vi "Check SLAM LM's.vi"(8 "error in (no error)":errorcluster, 10 "SLAM In":T2, 11 "Observed LM Array":T1(array[cluster])) -> (0 "error out":errorcluster, 2 "SLAM Out":T2, 3 "Observed LM Out":T1(array[cluster]))   [LabVIEW 2009]
uses:
  Controls/SLAM.ctl
  <vilib>/Analysis/Matrix/Datatypes/RealMatrix.ctl
  <vilib>/Analysis/Matrix/NI_Matrix.lvlib
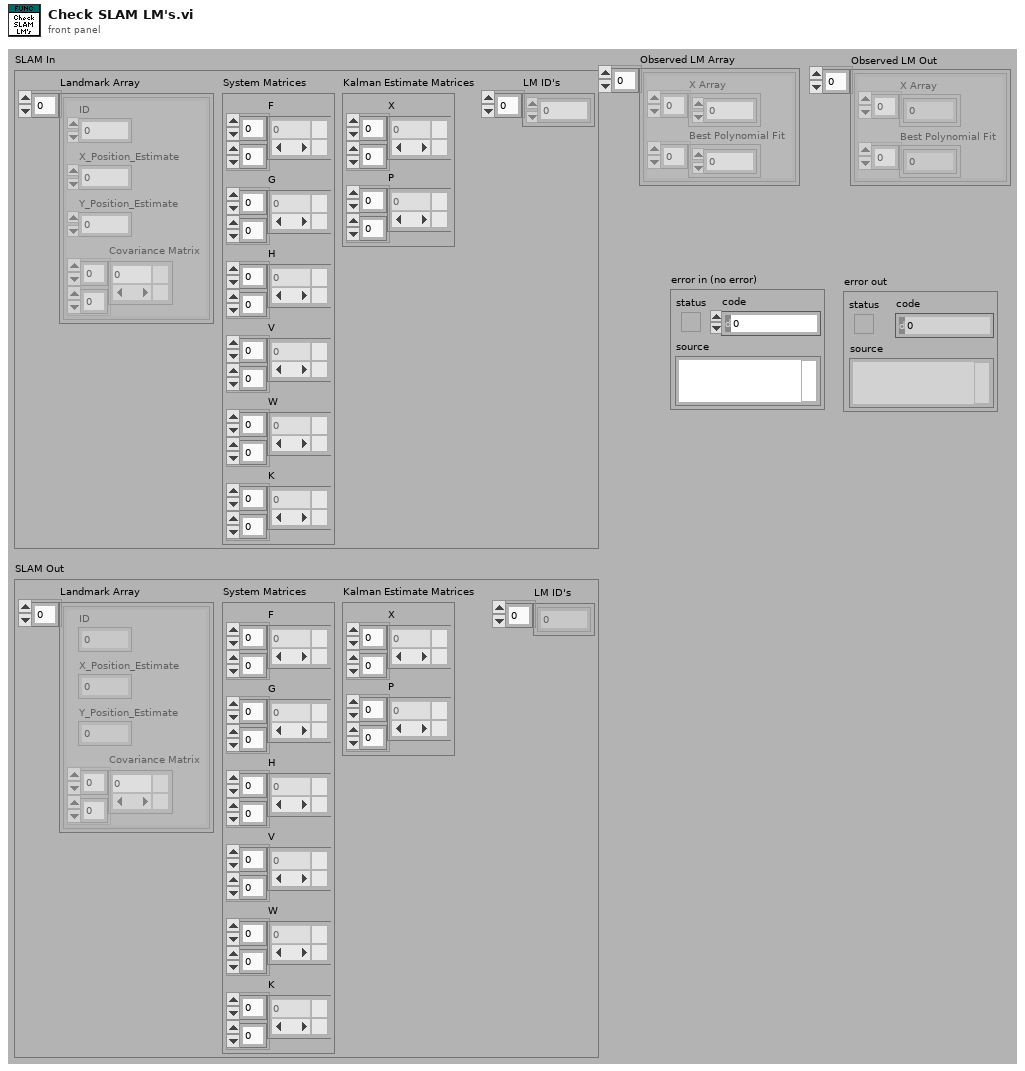
[diagram p1: front panel]
types:
  T1 = cluster{"X Array":dbl[], "Best Polynomial Fit":dbl[]}[]
  T2 = typedef "SLAM.ctl" = cluster{"Landmark Array":cluster{"ID":dbl, "X_Position_Estimate":dbl, "Y_Position_Estimate":dbl, "Covariance Matrix":T3}[], "System Matrices":cluster{"F":T3, "G":T3, "H":T3, "V":T3, "W":T3, "K":T3}, "Kalman Estimate Matrices":cluster{"X":T3, "P":T3}, "LM ID's":dbl[]}
  T3 = typedef "NI_Matrix.lvlib/RealMatrix.ctl" = dbl[][]
  T4 = cluster{"ID":dbl, "X_Position_Estimate":dbl, "Y_Position_Estimate":dbl, "Covariance Matrix":T3}[]
  T5 = cluster{"ID":dbl, "X_Position_Estimate":dbl, "Y_Position_Estimate":dbl, "Covariance Matrix":T3}
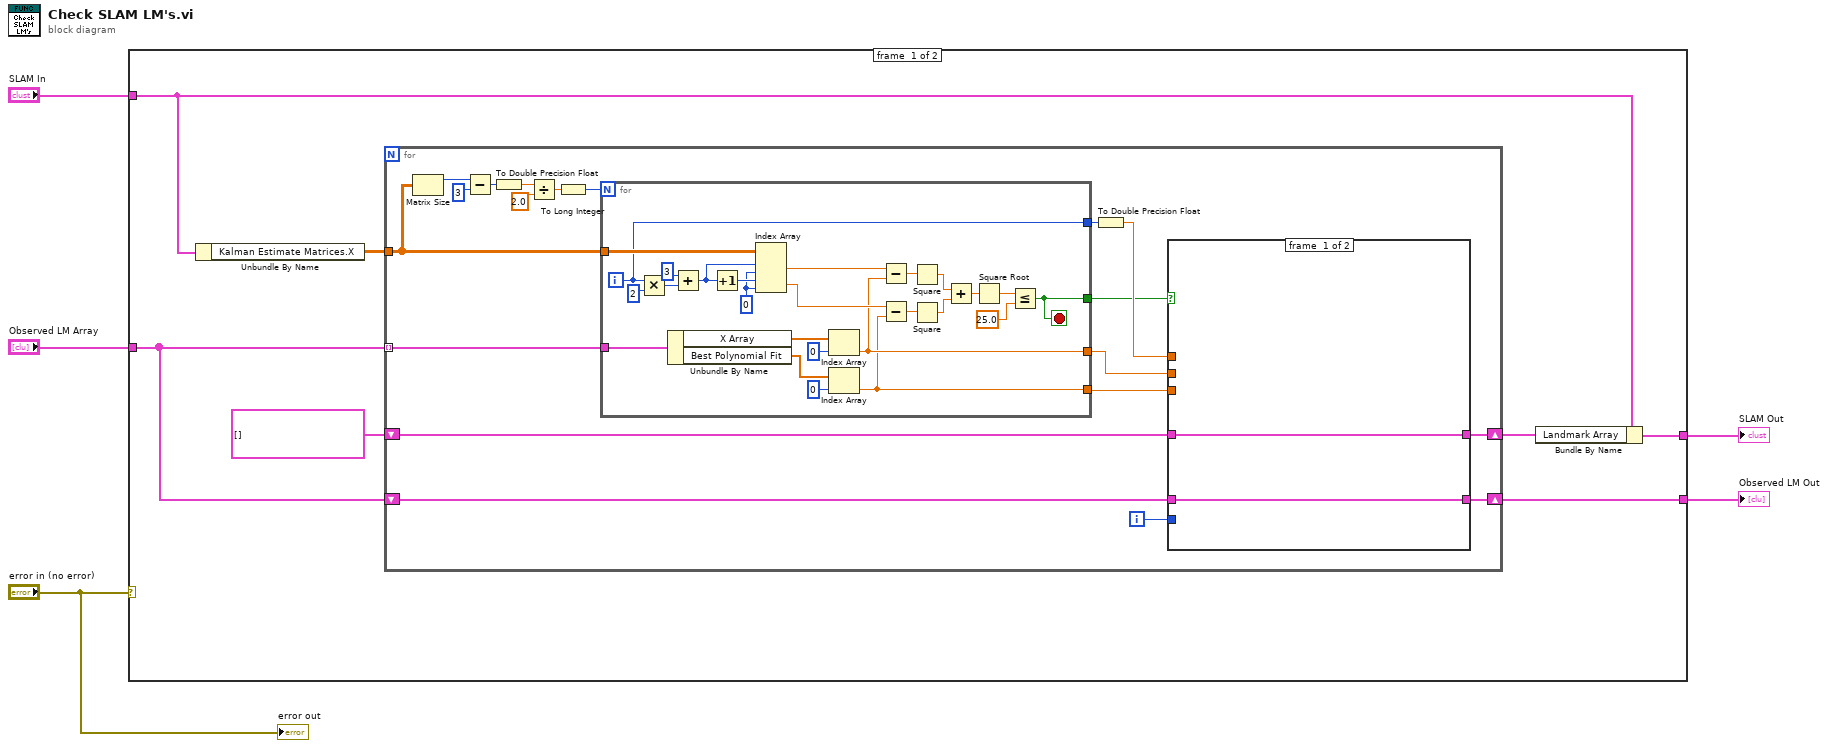
[diagram p0: block diagram]
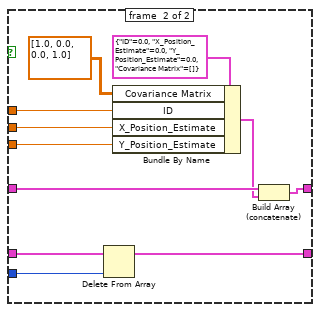
[diagram p2: hidden frame]
diagram:
  n1 = case shown="No Error" "error in (no error)" {
    tunnel: "SLAM In" -> [w11 _]
    tunnel: [w8 _] -> w4
    tunnel: "Observed LM Array" -> [w7 _]
    tunnel: [w6 _] -> w2
    frame #0 {
      n2 = Unbundle By Name(w11) -> ("Kalman Estimate Matrices.X"=w12:T3)
      n3 = for {
        tunnel: w7 -> [w31] mode=indexing
        tunnel: w12 -> [w23]
        shift-right: [w16] -> w9
        shift-left: T4 [] ("Landmark Array") -> [w17]
        shift-right: [w13] -> w6
        shift-left: w7 -> [w15]
        i -> [w14]
        n4 = Matrix Size(0:w23) -> (1:w30:i32)  [unwired: 1 out]
        n5 = Subtract(x=w30, y=3) -> (x-y=w28:i32)
        n6 = To Double Precision Float(number=w28) -> (double precision float=w27:dbl)
        n7 = Divide(x=w27, y=2.0) -> (x/y=w25:dbl)
        n8 = To Long Integer(number=w25) -> (32bit integer=w24:i32)
        n9 = for {
          N: w24 -> [_]
          tunnel: w31 -> [w58]
          tunnel: [w57] -> w18
          tunnel: w23 -> [w48]
          tunnel: [w47] -> w22
          tunnel: [w46] -> w21
          tunnel: [w45] -> w20
          i -> [w45]
          stop <- w57 stop-if-true
          w51 = 0 ("index (col)")
          n10 = Multiply(x=w45, y=2) -> (x*y=w55:i32)
          n11 = Unbundle By Name(w58) -> ("X Array"=w61:dbl[], "Best Polynomial Fit"=w62:dbl[])
          n12 = Add(x=3, y=w55) -> (x+y=w53:i32)
          n13 = Increment(x=w53) -> (x+1=w52:i32)
          n14 = Index Array(array=w48, index (row) #1=w53, index (col) #1=w51, index (row) #2=w52, index (col) #2=w51) -> (element #1=w50:dbl, element #2=w49:dbl)
          n15 = Index Array(array=w61, index=0) -> (element=w47:dbl)
          n16 = Index Array(array=w62, index=0) -> (element=w46:dbl)
          n17 = Subtract(x=w50, y=w47) -> (x-y=w68:dbl)
          n18 = Subtract(x=w49, y=w46) -> (x-y=w69:dbl)
          n19 = Square(x=w68) -> (x^2=w67:dbl)
          n20 = Square(x=w69) -> (x^2=w66:dbl)
          n21 = Add(x=w67, y=w66) -> (x+y=w65:dbl)
          n22 = Square Root(x=w65) -> (sqrt(x)=w64:dbl)
          n23 = Less Or Equal?(x=w64, y=25.0) -> (x <= y?=w57:bool)
        }
        n24 = To Double Precision Float(number=w20) -> (double precision float=w19:dbl)
        n25 = case shown="True" w18 {
          tunnel: w22 -> [_ w43]
          tunnel: w21 -> [_ w42]
          tunnel: w19 -> [_ w41]
          tunnel: w17 -> [w33 w40]
          tunnel: [w33 w38] -> w16
          tunnel: w15 -> [w32 w37]
          tunnel: w14 -> [_ w36]
          tunnel: [w32 w35] -> w13
          frame #0 {
          }
          frame #1 {
            n26 = Delete From Array(array=w37, index=w36) -> (array with subset deleted=w35:T1)  [unwired: 1 in, 1 out]
            n27 = Bundle By Name(cluster=T5 {"ID"=0.0, "X_Position_Estimate"=0.0, "Y_Position_Estimate"=0.0, "Covariance Matrix"=[]} ("Landmarks"), "Covariance Matrix"=T3 [[1.0, 0.0], [0.0, 1.0]], "ID"=w41, "X_Position_Estimate"=w43, "Y_Position_Estimate"=w42) -> (w39:T5)
            n28 = Build Array (concatenate)(w40, w39) -> (w38:T4)
          }
        }
      }
      n29 = Bundle By Name(cluster=w11, "Landmark Array"=w9) -> (w8:T2)
    }
    frame #1 {
    }
  }
  "SLAM Out" <- w4
  "Observed LM Out" <- w2
  "error out" <- "error in (no error)"
